vi "wait on clock.vi"(8 "error in":errorcluster, 11 "timing source in":refnum<class "scan engine timing source.lvclass">) -> (0 "error out":errorcluster, 2 "ticks since last call":u32, 3 "timing source out":refnum<class "scan engine timing source.lvclass">)   [LabVIEW 2013, in "scan engine timing source.lvclass"]
doc: "This core timing function is used inside of a loop to wait for a clock signal, or dt ticks of a clock signal."
uses:
  scan engine timing source.lvclass
  timing source/TBM timing source.lvclass/TBM timing source.ctl
  timing source/TBM timing source.lvclass
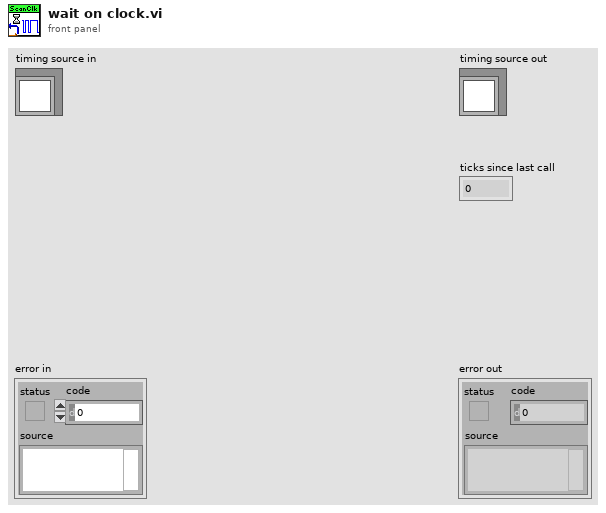
[diagram p1: front panel]
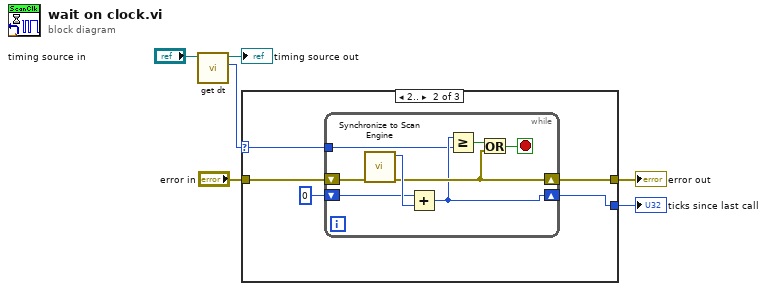
[diagram p0: block diagram]
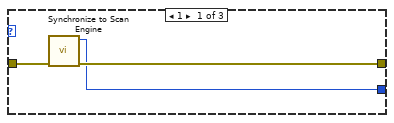
[diagram p2: hidden frame]
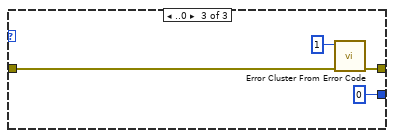
[diagram p3: hidden frame]
diagram:
  n1 = call "get dt.vi"("timing source in"="timing source in") -> ("dt"=w4:u32, "timing source out"=→"timing source out":refnum<class "scan engine timing source.lvclass">)  [unwired: 9 in]
  n2 = case shown="2.." w4 {
    selector: w4 -> [_ w10 _]
    tunnel: "error in" -> [w9 w14 w26]
    tunnel: [w8 w13 w24] -> w2
    tunnel: [w7 w11 u32 0 ("scans since last call")] -> w1
    frame 1 {
      n3 = call <vilib>:"Synchronize to Scan Engine.vi"("error in (no error)"=w9) -> ("error out"=w8:errorcluster, "scans since last call"=w7:u32)  [unwired: 9 in]
    }
    frame 2.. {
      n4 = while {
        shift-right: [w18] -> w13
        shift-left: w14 -> [w22]
        shift-right: [w17] -> w11
        shift-left: u32 0 ("scans since last call") -> [w20]
        tunnel: w10 -> [w16]
        stop <- w19 stop-if-true
        n5 = call <vilib>:"Synchronize to Scan Engine.vi"("error in (no error)"=w22) -> ("error out"=w18:errorcluster, "scans since last call"=w21:u32)  [unwired: 9 in]
        n6 = Add(x=w20, y=w21) -> (x+y=w17:u32)
        n7 = Greater Or Equal?(x=w17, y=w16) -> (x >= y?=w15:bool)
        n8 = Or(x=w15, y=w18) -> (x .or. y?=w19:bool)
      }
    }
    frame ..0 {
      n9 = call <vilib>:"Error Cluster From Error Code.vi"("error in (no error)"=w26, "error code (0)"=1) -> ("error out"=w24:errorcluster)  [unwired: 7 in]
    }
  }
  "error out" <- w2
  "ticks since last call" <- w1
